vi "Read Snap Measurement.vi"(8 "error in":errorcluster, 10 "Trigger_Start":timestamp, 11 "3300 in":refnum<class "3300.lvclass">) -> (0 "error out":errorcluster, 2 "Snapshot Data":waveform(dbl)[](array[waveform]), 3 "3300 out":refnum<class "3300.lvclass">)   [LabVIEW 2019, in "3300.lvlib" / "3300.lvclass"]
uses:
  Library/3300.lvclass
  C:/Users/Public/Documents/Development/builds/Instruments/Electronic Load.lvlibp/Library/Electronic Load.lvclass
  C:/Users/Public/Documents/Development/builds/Engine/Monitored Actor.lvlibp/Monitored Actor/Monitored Actor/Monitored Actor.lvclass
  C:/Users/Public/Documents/Development/builds/Instruments/Instruments.lvlibp/Library/Instruments.lvclass
  builds/Instruments/Electronic Load.lvlibp/Accessors/Read Available Channels.vi
  builds/Instruments/Electronic Load.lvlibp/Private/GUI/Read Channel_Names.vi
  builds/Engine/Monitored Actor.lvlibp/Monitored Actor/Monitored Actor/Read Actor Label.vi
  builds/Instruments/Instruments.lvlibp/Accessors/Read dt.vi
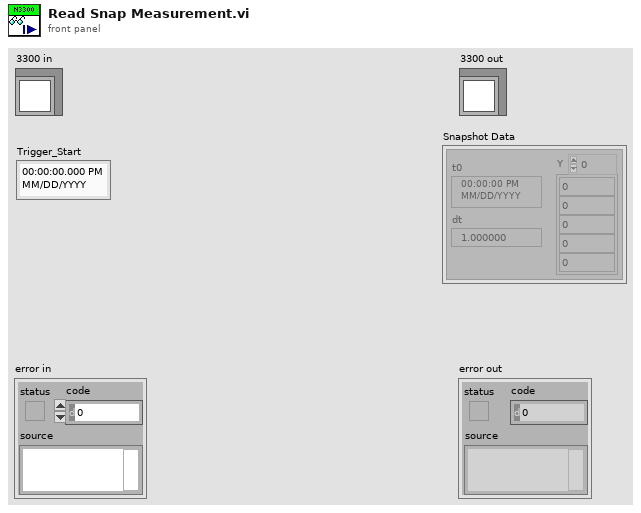
[diagram p1: front panel]
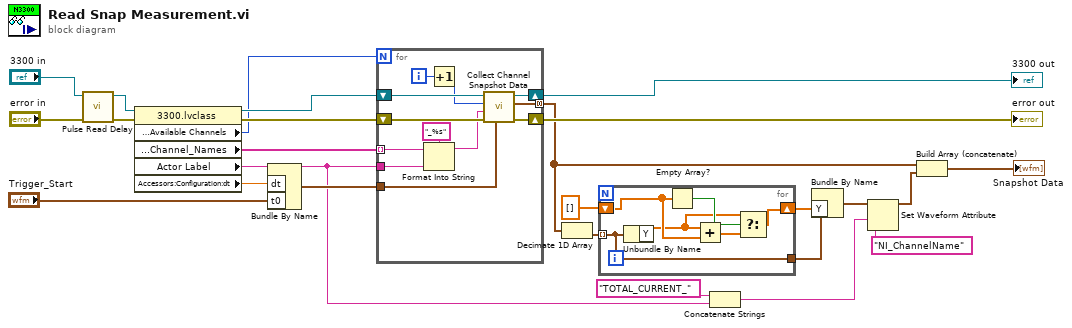
[diagram p0: block diagram]
diagram:
  n1 = call "Pulse Read Delay.vi"("error in (no error)"="error in", "3300 in"="3300 in") -> ("error out"=w3:errorcluster, "3300 out"=w2:refnum<class "3300.lvclass">)  [unwired: 8 in]
  n2 = property class="3300.lvclass"(reference=w2, error in=w3) -> (reference out=w25:refnum<class "3300.lvclass">, error out=w24:errorcluster, "Accessors:Configuration:Available Channels"=w1:i32, "Protected:Accessors:GUI:Channel_Names"=w21:string[], "Actor Label"=w7:string, "Accessors:Configuration:dt"=w20:dbl)
  n3 = Bundle By Name("dt"=w20, "t0"="Trigger_Start") -> (w22:waveform(dbl))  [unwired: 1 in]
  n4 = for {
    N: w1 -> [_]
    shift-right: [w33] -> w19
    shift-left: w25 -> [w36]
    shift-right: [w32] -> w14
    shift-left: w24 -> [w37]
    tunnel: w22 -> [w31]
    tunnel: w21 -> [w29] mode=indexing
    tunnel: w7 -> [w30]
    tunnel: [w26] -> w12 mode=concatenating
    i -> [w35]
    n5 = Format Into String(format string="_%s", initial string=w29, w30) -> (resulting string=w28:string)  [unwired: 1 in, 1 out]
    n6 = Increment(x=w35) -> (x+1=w34:i32)
    n7 = call "Collect Channel Snapshot Data.vi"("Template waveform"=w31, "error in"=w37, "Channel Name"=w28, "Channel"=w34, "3300 in"=w36) -> ("error out"=w32:errorcluster, "Channel Data"=w26:waveform(dbl)[], "3300 out"=w33:refnum<class "3300.lvclass">)  [unwired: 4 in]
  }
  "error out" <- w14
  "3300 out" <- w19
  n8 = Decimate 1D Array(w12) -> (w18:waveform(dbl)[])  [unwired: 1 out]
  n9 = for {
    tunnel: w18 -> [w38] mode=indexing
    shift-right: [w40] -> w15
    shift-left: dbl[] [] -> [w42]
    tunnel: [w38] -> w16
    n10 = Unbundle By Name(w38) -> ("Y"=w41:dbl[])
    n11 = Empty Array?(array=w42) -> (empty?=w43:bool)
    n12 = Add(x=w41, y=w42) -> (x+y=w39:dbl[])
    n13 = Select(t=w41, s=w43, f=w39) -> (s? t:f=w40:dbl[])
  }
  n14 = Concatenate Strings("TOTAL_CURRENT_" ("string"), w7) -> (w6:string)
  n15 = Bundle By Name(cluster=w16, "Y"=w15) -> (w13:waveform(dbl))
  n16 = Set Waveform Attribute(5:w6, 6:"NI_ChannelName" ("name"), 7:w13) -> (3:w10:waveform(dbl))  [unwired: 1 in, 2 out]
  n17 = Build Array (concatenate)(w12, w10) -> (→"Snapshot Data":waveform(dbl)[])
